vi "vipm_ExitVIPM.vi"(8 "error in (no error)":errorcluster, 11 "CommandLine":string[](array[string])) -> (0 "error out":errorcluster, 2 "test details":string, 3 "output to action":string)   [LabVIEW 2014]
uses:
  _lvcicd/_lvcicd_support_2014.lvlib
  <vilib>/JKI/VIPM API/VIPM API_vipm_api.lvlib
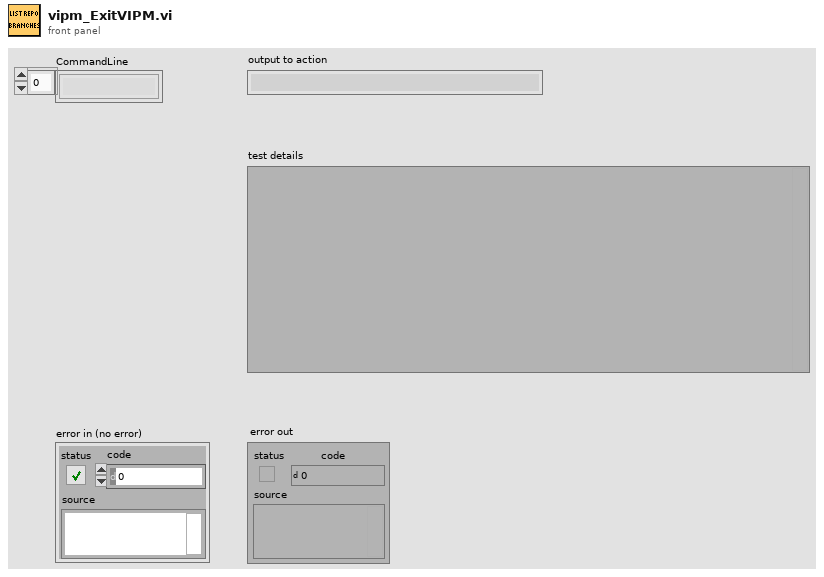
[diagram p1: front panel]
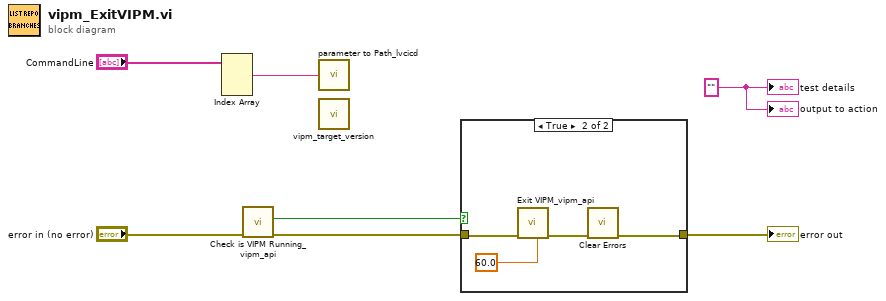
[diagram p0: block diagram]
diagram:
  w4 = "" ("test details")
  n1 = Index Array(array="CommandLine") -> (element #1=w6:string)  [unwired: 3 in, 2 out]
  n2 = call <vilib>:"Check is VIPM Running_vipm_api.vi"("error in (no error)"="error in (no error)") -> ("error out"=w5:errorcluster, "is Running"=w2:bool)  [unwired: 9 in]
  n3 = call "parameter to Path_lvcicd.vi"("String"=w6) -> ()  [unwired: 1 out]
  n4 = call "vipm_target_version.vi"() -> ()  [unwired: 11 in, 1 out]
  n5 = case shown="True" w2 {
    tunnel: w5 -> [w8 w12]
    tunnel: [w8 w9] -> w1
    frame False {
    }
    frame True {
      n6 = call <vilib>:"Exit VIPM_vipm_api.vi"("Timeout in seconds (0: no timeout)"=60.0, "error in (no error)"=w12) -> ("error out"=w11:errorcluster)  [unwired: 9 in]
      n7 = call <vilib>:"Clear Errors.vi"("error in (no error)"=w11) -> ("error out"=w9:errorcluster)  [unwired: 5 in, 1 out]
    }
  }
  "error out" <- w1
  "test details" <- w4
  "output to action" <- w4
